vi "Write shared variable refnum out.vi"(8 "error in (no error)":errorcluster, 10 "shared variable refnum out":refnum<k21>, 11 "ibsen in":refnum<class "ibsen.lvclass">) -> (0 "error out":errorcluster, 3 "ibsen out":refnum<class "ibsen.lvclass">)   [LabVIEW 2019, in "ibsen.lvlib" / "ibsen.lvclass"]
uses:
  ibsen.lvclass
  ibsen.lvclass/ibsen.ctl
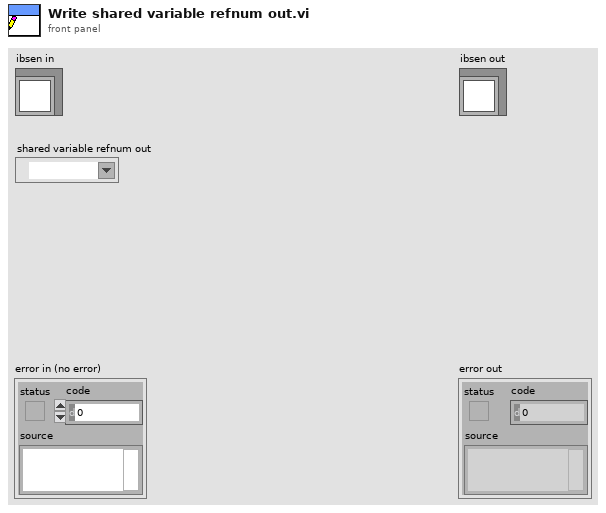
[diagram p1: front panel]
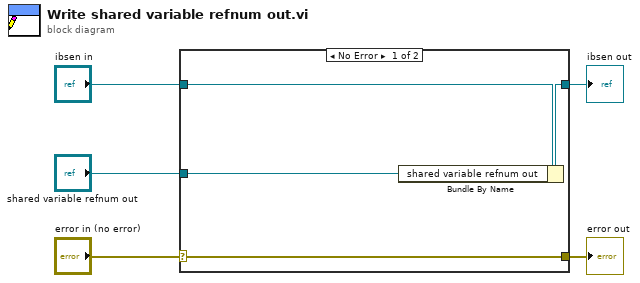
[diagram p0: block diagram]
diagram:
  n1 = case shown="No Error" "error in (no error)" {
    selector: "error in (no error)" -> [w9 w10]
    tunnel: [w9 w10] -> w4
    tunnel: [w7 w11] -> w2
    tunnel: "ibsen in" -> [w8 w11]
    tunnel: "shared variable refnum out" -> [w6 _]
    frame No Error {
      n2 = Bundle By Name(cluster=w8, "shared variable refnum out"=w6) -> (w7:refnum<class "ibsen.lvclass">)
    }
    frame Error {
    }
  }
  "error out" <- w4
  "ibsen out" <- w2
